vi "(SubVI)Calculate DNA geometry of Length and Force For Passive Force Clamp_YCC.vi"(6 "trap height(nm)":dbl, 7 "bead radius(nm)":dbl=515.0, 8 "Start point of Xbd for pFC (nm)":dbl, 10 "Xst (nm)":dbl[](array[numeric]), 11 "Xbd (nm)":dbl[](array[numeric])) -> (0 "zbd (nm)":dbl[](array[numeric]), 2 "xDNA (nm)":dbl[](array[numeric]), 4 "Check Xbd for pFC (nm)":dbl)   [LabVIEW 2014]
panel:
  out "Zbd pFC (nm)":dbl
  in  "Focal shift factor":dbl=1.22
  in  "kx/kz":dbl=3.5
  out "Fx":dbl
  out "Force (pN)":dbl[](array[numeric])
  in  "Force constant (pN/nm)":dbl=0.0154
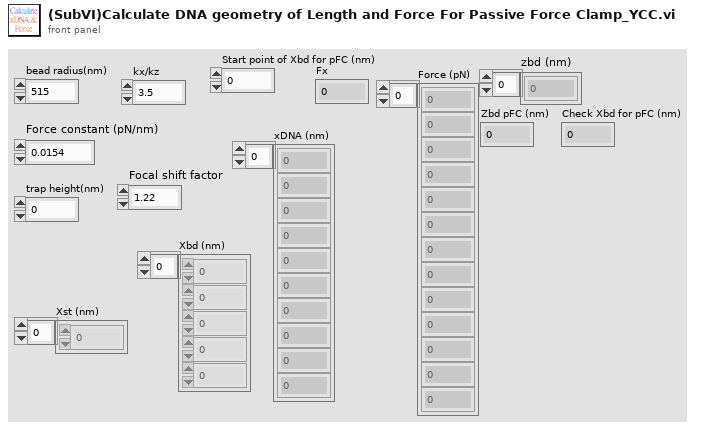
[diagram p1: front panel]
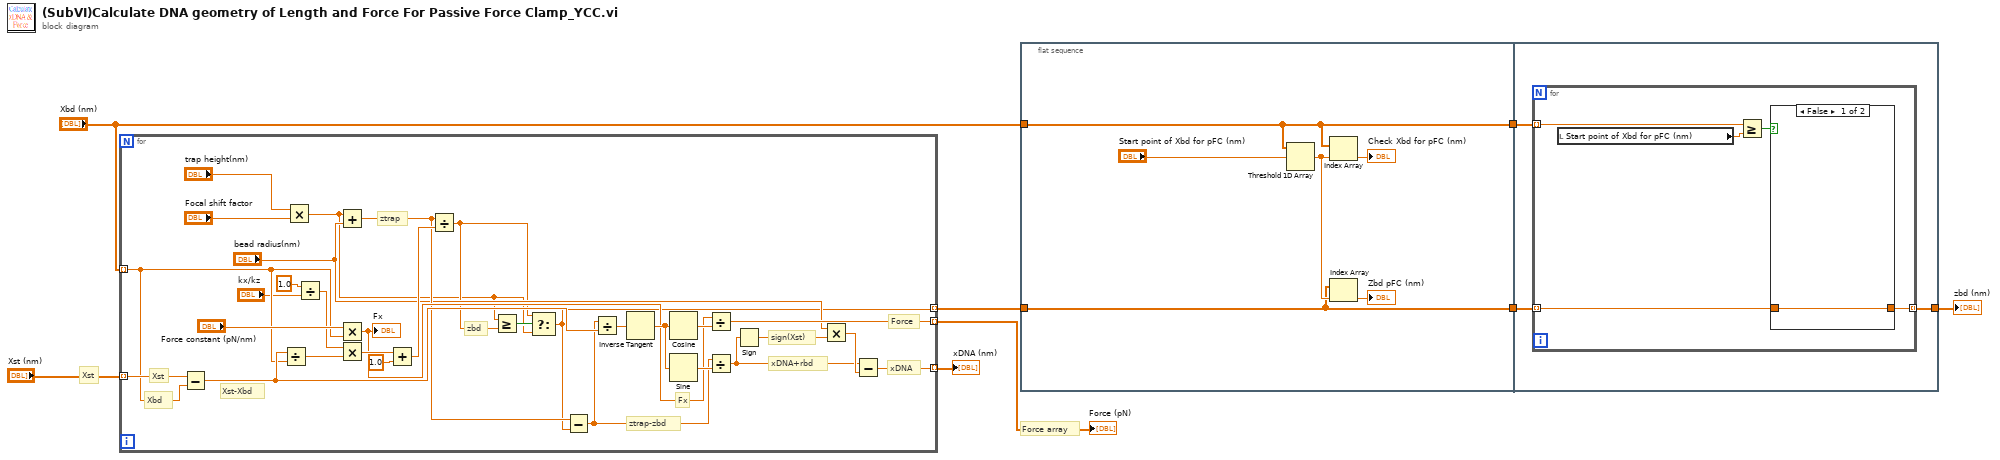
[diagram p0: block diagram]
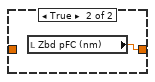
[diagram p2: hidden frame]
diagram:
  # "Force array"
  # "Xst"
  n1 = for {
    tunnel: "Xst (nm)" -> [w27] mode=indexing
    tunnel: "Xbd (nm)" -> [w22] mode=indexing
    tunnel: [w26] -> w7 mode=indexing
    tunnel: [w25] -> w8 mode=indexing
    tunnel: [w10] -> w4 mode=indexing
    # "ztrap"
    # "xDNA"
    # "xDNA+rbd"
    # "Force"
    # "Fx"
    # "sign(Xst)"
    # "ztrap-zbd"
    # "Xst-Xbd"
    # "zbd"
    # "Xst"
    # "Xbd"
    n2 = Subtract(x=w27, y=w22) -> (x-y=w34:dbl)
    n3 = Divide(x=w34, y=w22) -> (x/y=w38:dbl)
    n4 = Multiply(x="trap height(nm)", y="Focal shift factor") -> (x*y=w9:dbl)
    n5 = Divide(x=1.0, y="kx/kz") -> (x/y=w19:dbl)
    n6 = Add(x=w9, y="bead radius(nm)") -> (x+y=w15:dbl)
    n7 = Multiply(x="Force constant (pN/nm)", y=w22) -> (x*y=w21:dbl)
    "Fx" <- w21
    n8 = Multiply(x=w19, y=w38) -> (x*y=w36:dbl)
    n9 = Add(x=w36, y=1.0) -> (x+y=w35:dbl)
    n10 = Divide(x=w15, y=w35) -> (x/y=w11:dbl)
    n11 = Greater Or Equal?(x=w9, y=w11) -> (x >= y?=w14:bool)
    n12 = Select(t=w11, s=w14, f=w9) -> (s? t:f=w10:dbl)
    n13 = Subtract(x=w15, y=w10) -> (x-y=w12:dbl)
    n14 = Divide(x=w12, y=w34) -> (x/y=w33:dbl)
    n15 = Inverse Tangent(1:w33) -> (0:w31:dbl)
    n16 = Cosine(x=w31) -> (cos(x)=w30:dbl)
    n17 = Sine(x=w31) -> (sin(x)=w32:dbl)
    n18 = Divide(x=w21, y=w30) -> (x/y=w25:dbl)
    n19 = Divide(x=w12, y=w32) -> (x/y=w24:dbl)
    n20 = Sign(1:w24) -> (0:w29:dbl)
    n21 = Multiply(x="bead radius(nm)", y=w29) -> (x*y=w28:dbl)
    n22 = Subtract(x=w24, y=w28) -> (x-y=w26:dbl)
  }
  "Force (pN)" <- w8
  "xDNA (nm)" <- w7
  n23 = flat-sequence {
    tunnel: "Xbd (nm)" -> [w39]
    tunnel: w4 -> [w40]
    tunnel: [w40] -> w3
    tunnel: [w39] -> w2
    tunnel: w3 -> [w47]
    tunnel: w2 -> [w46]
    tunnel: [w45] -> w1
    frame #0 {
      n24 = Threshold 1D Array(2:"Start point of Xbd for pFC (nm)", 3:w39) -> (0:w42:dbl)  [unwired: 1 in]
      n25 = Index Array(array=w39, index=w42) -> (element=→"Check Xbd for pFC (nm)":dbl)
      n26 = Index Array(array=w40, index=w42) -> (element=→"Zbd pFC (nm)":dbl)
    }
    frame #1 {
      n27 = for {
        tunnel: w47 -> [w52] mode=indexing
        tunnel: [w51] -> w45 mode=indexing
        tunnel: w46 -> [w50] mode=indexing
        n28 = local read "Start point of Xbd for pFC (nm)"() -> (w49:dbl)
        n29 = Greater Or Equal?(x=w50, y=w49) -> (x >= y?=w48:bool)
        n30 = case shown="False" w48 {
          tunnel: w52 -> [w53 _]
          tunnel: [w53 w54] -> w51
          frame False {
          }
          frame True {
            n31 = local read "Zbd pFC (nm)"() -> (w54:dbl)
          }
        }
      }
    }
  }
  "zbd (nm)" <- w1
